vi "CheckDeviceStatusForBootSequence.vi"(2 "error in":errorcluster) -> (17 "error out":errorcluster)   [LabVIEW 2011]
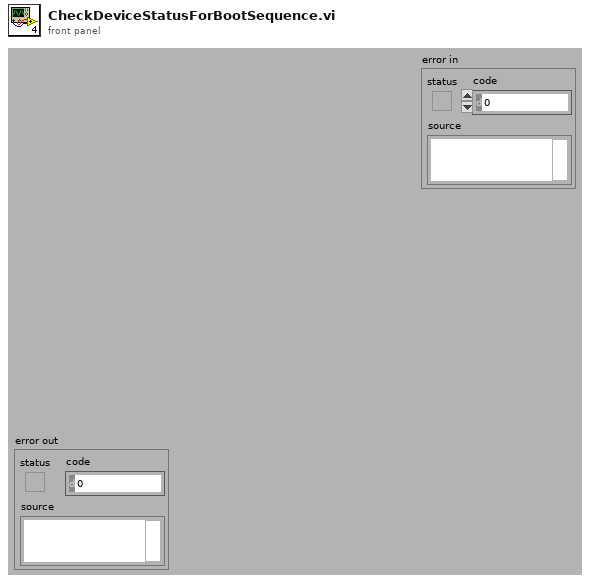
[diagram p1: front panel]
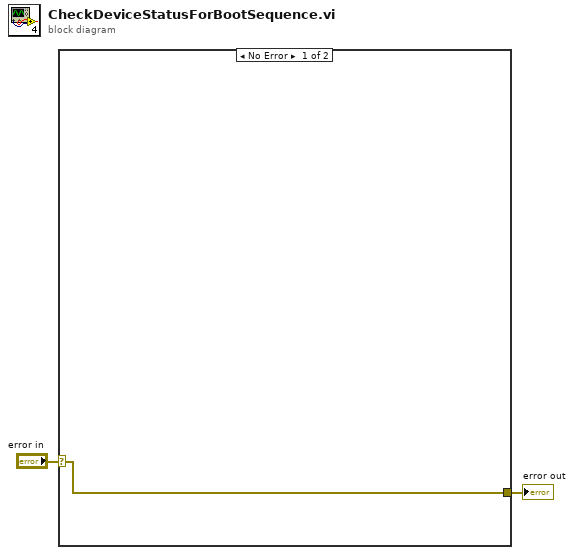
[diagram p0: block diagram]
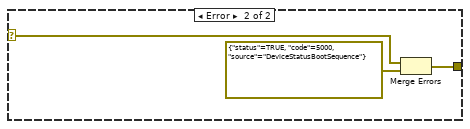
[diagram p2: hidden frame]
diagram:
  n1 = case shown="No Error" "error in" {
    selector: "error in" -> [w3 w6]
    tunnel: [w3 w4] -> w1
    frame No Error {
    }
    frame Error {
      n2 = Merge Errors(w6, errorcluster {"status"=TRUE, "code"=5000, "source"="DeviceStatusBootSequence"} ("error out")) -> (w4:errorcluster)
    }
  }
  "error out" <- w1
